vi "anott. visibility and colour.vi"(8 "error in (no error)":errorcluster, 9 "Annotation No":i32, 10 "Name Visible":bool, 11 "XYGraph in":refnum<vi>) -> (0 "error out":errorcluster, 3 "XYGraph out":refnum<vi>)   [LabVIEW 2014]
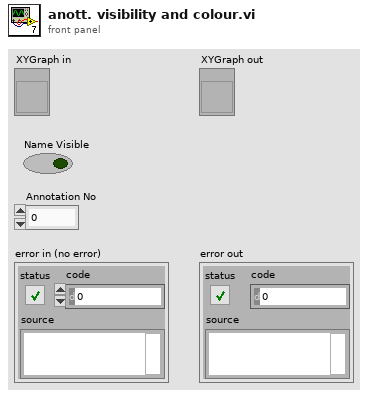
[diagram p1: front panel]
types:
  T1 = typedef "LVAnnotationListTypeDef.ctl" = cluster{"Name":string, "Color":u32, "Style":u8, "Point Style":u8, "Name Visible":bool, "Allow Drag":bool, "Annotation Mode":u32, "Plot":i32, "Index":i32, "Position":cluster{"X":dbl, "Y":dbl}, "X Scale":u32, "Y Scale":u32, "Show Arrow":bool, "Lock Name":bool, "Plot Area":i32, "Label Offset":cluster{"X":dbl, "Y":dbl}}[]
  T2 = cluster{"Name":string, "Color":u32, "Style":u8, "Point Style":u8, "Name Visible":bool, "Allow Drag":bool, "Annotation Mode":u32, "Plot":i32, "Index":i32, "Position":cluster{"X":dbl, "Y":dbl}, "X Scale":u32, "Y Scale":u32, "Show Arrow":bool, "Lock Name":bool, "Plot Area":i32, "Label Offset":cluster{"X":dbl, "Y":dbl}}
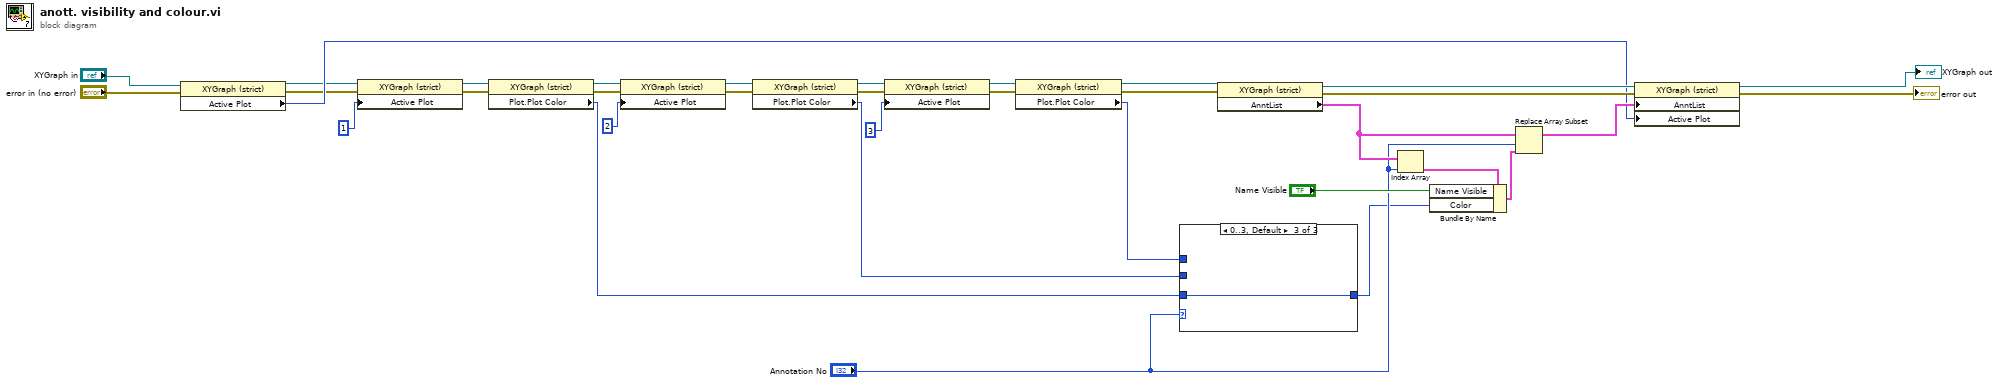
[diagram p0: block diagram]
diagram:
  n1 = property class="XYGraph (strict)"(reference="XYGraph in", error in="error in (no error)") -> (reference out=w13:refnum<vi>, error out=w14:errorcluster, "Active Plot"=w25:u32)
  n2 = property class="XYGraph (strict)"(reference=w13, error in=w14, "Active Plot"=u32 1) -> (reference out=w21:refnum<vi>, error out=w22:errorcluster)
  n3 = property class="XYGraph (strict)"(reference=w21, error in=w22) -> (reference out=w18:refnum<vi>, error out=w11:errorcluster, "Plot.Plot Color"=w7:u32)
  n4 = property class="XYGraph (strict)"(reference=w18, error in=w11, "Active Plot"=u32 2) -> (reference out=w24:refnum<vi>, error out=w23:errorcluster)
  n5 = property class="XYGraph (strict)"(reference=w24, error in=w23) -> (reference out=w16:refnum<vi>, error out=w17:errorcluster, "Plot.Plot Color"=w4:u32)
  n6 = property class="XYGraph (strict)"(reference=w16, error in=w17, "Active Plot"=u32 3) -> (reference out=w19:refnum<vi>, error out=w20:errorcluster)
  n7 = property class="XYGraph (strict)"(reference=w19, error in=w20) -> (reference out=w6:refnum<vi>, error out=w5:errorcluster, "Plot.Plot Color"=w3:u32)
  n8 = case shown="0..3, Default" "Annotation No" {
    tunnel: [w35 w36 w37] -> w8
    tunnel: w7 -> [_ _ w37]
    tunnel: w4 -> [w35 _ _]
    tunnel: w3 -> [_ w36 _]
    frame 4..7 {
    }
    frame 8..11 {
    }
    frame 0..3, Default {
    }
  }
  n9 = property class="XYGraph (strict)"(reference=w6, error in=w5) -> (reference out=w31:refnum<vi>, error out=w30:errorcluster, "AnntList"=w28:T1)
  n10 = Index Array(array=w28, index="Annotation No") -> (element=w32:T2)
  n11 = Bundle By Name(cluster=w32, "Name Visible"="Name Visible", "Color"=w8) -> (w33:T2)
  n12 = Replace Array Subset "Replace Array Subset"(array=w28, new element=w33, index="Annotation No") -> (w29:T1)
  n13 = property class="XYGraph (strict)"(reference=w31, error in=w30, "AnntList"=w29, "Active Plot"=w25) -> (reference out=→"XYGraph out":refnum<vi>, error out=→"error out":errorcluster)
